vi "Is VI Front Panel Open.vi"(8 "error in (no error)":errorcluster, 10 "VI Name":string, 11 "App Ref":refnum<vi>) -> (0 "error out":errorcluster, 3 "Front Panel Open?":bool)   [LabVIEW 2020, in "MacroAssert.lvlib"]
doc: "Checks if a VI front panel is open by first checking the VI itself, and also checking any open clones if the VI is reentrant."
uses:
  MacroAssert.lvlib
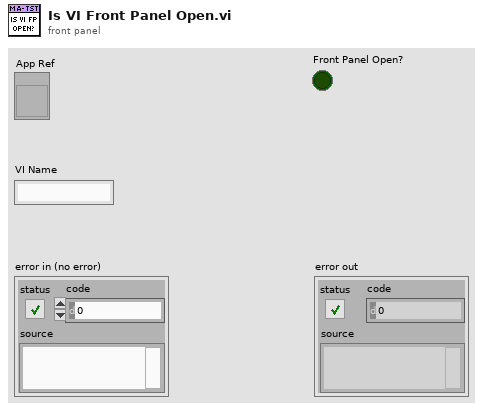
[diagram p1: front panel]
types:
  T1 = enum32{"Invalid", "Standard", "Closed", "Hidden", "Minimized", "Maximized"}[]
  T2 = enum32{"Invalid", "Standard", "Closed", "Hidden", "Minimized", "Maximized"}
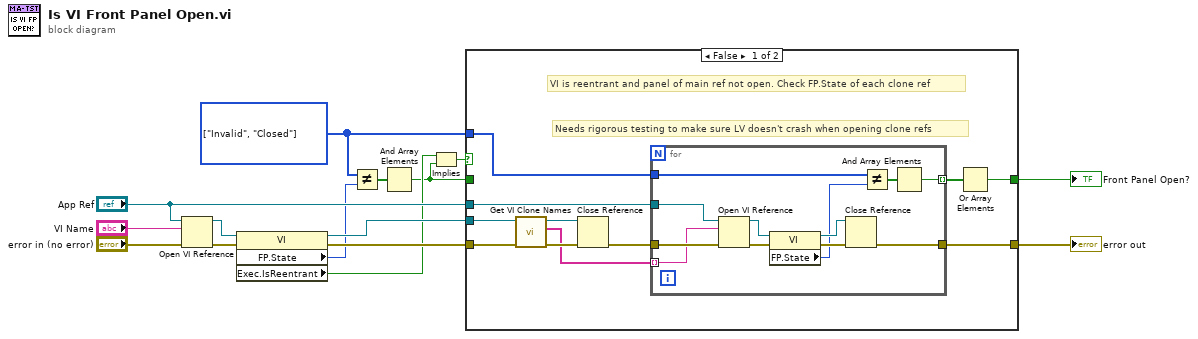
[diagram p0: block diagram]
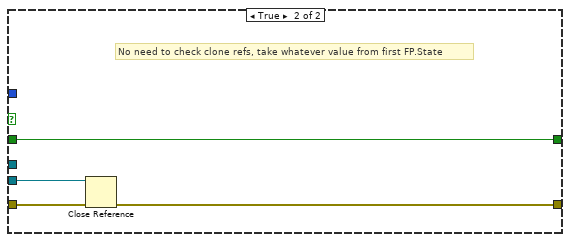
[diagram p2: hidden frame]
diagram:
  w4 = T1 [enum."Invalid", enum."Closed"] items=["Invalid", "Standard", "Closed", "Hidden", "Minimized", "Maximized"]
  n1 = Open VI Reference(application reference (local)="App Ref", vi path="VI Name", error in (no error)="error in (no error)") -> (vi reference=w11:refnum<vi>, error out=w14:errorcluster)  [unwired: 3 in]
  n2 = property class="VI"(reference=w11, error in=w14) -> (reference out=w10:refnum<vi>, error out=w13:errorcluster, "FP.State"=w8:T2, "Exec.IsReentrant"=w3:bool)
  n3 = Not Equal?(x=w4, y=w8) -> (x != y?=w7:bool[])
  n4 = And Array Elements(Boolean array=w7) -> (logical AND=w1:bool)
  n5 = Implies(1:w1, 2:w3) -> (0:w2:bool)
  n6 = case shown="False" w2 {
    tunnel: w13 -> [w26 w42]
    tunnel: w10 -> [w22 w40]
    tunnel: [w23 w41] -> w12
    tunnel: [w16 w39] -> w5
    tunnel: w4 -> [w18 _]
    tunnel: "App Ref" -> [w20 _]
    tunnel: w1 -> [_ w39]
    frame False {
      # "VI is reentrant and panel of main ref not open. Check FP.State of each clone ref"
      # "Needs rigorous testing to make sure LV doesn't crash when opening clone refs"
      n7 = call "Get VI Clone Names.vi"("error in (no error)"=w26, "VI Ref"=w22) -> ("error out"=w25:errorcluster, "Clone Names"=w19:string[], "VI Ref out"=w21:refnum<vi>)  [unwired: 7 in]
      n8 = Close Reference(reference=w21, error in (no error)=w25) -> (error out=w24:errorcluster)
      n9 = for {
        tunnel: w24 -> [w37]
        tunnel: w19 -> [w30] mode=indexing
        tunnel: [w35] -> w23
        tunnel: w18 -> [w28]
        tunnel: [w27] -> w17 mode=indexing
        tunnel: w20 -> [w32]
        n10 = Open VI Reference(application reference (local)=w32, vi path=w30, error in (no error)=w37) -> (vi reference=w34:refnum<vi>, error out=w38:errorcluster)  [unwired: 3 in]
        n11 = property class="VI"(reference=w34, error in=w38) -> (reference out=w33:refnum<vi>, error out=w36:errorcluster, "FP.State"=w29:T2)
        n12 = Close Reference(reference=w33, error in (no error)=w36) -> (error out=w35:errorcluster)
        n13 = Not Equal?(x=w28, y=w29) -> (x != y?=w31:bool[])
        n14 = And Array Elements(Boolean array=w31) -> (logical AND=w27:bool)
      }
      n15 = Or Array Elements(Boolean array=w17) -> (logical OR=w16:bool)
    }
    frame True {
      # "No need to check clone refs, take whatever value from first FP.State"
      n16 = Close Reference(reference=w40, error in (no error)=w42) -> (error out=w41:errorcluster)
    }
  }
  "error out" <- w12
  "Front Panel Open?" <- w5
